vi "Write Error to System Log.vi"(6 "log each error instance (F)":bool, 8 "error in":errorcluster, 10 "message":string, 11 "identifier":string) -> (0 "error out":errorcluster)   [LabVIEW 2020, in "Ballard MIL-STD-1553 Engine.lvlib" / "Custom Device.lvlib"]
uses:
  ca55ed61-c1f5-4d13-8aef-490b87d2cf89.vi
  Custom Device.lvlib
  <vilib>/NI VeriStand/Custom Device Tools/Custom Device Utility Library/Custom Device Utility Library.lvlib
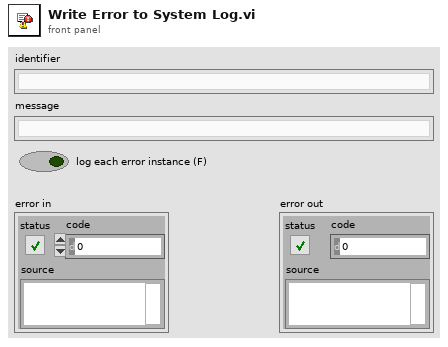
[diagram p1: front panel]
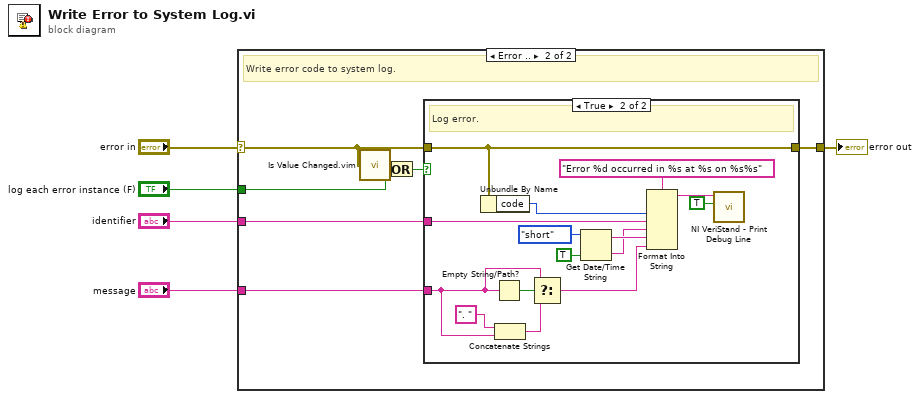
[diagram p0: block diagram]
diagram:
  n1 = case shown="Error .." "error in" {
    selector: "error in" -> [w6 w12]
    tunnel: [w6 w13] -> w5
    tunnel: "log each error instance (F)" -> [_ w9]
    tunnel: "identifier" -> [_ w8]
    tunnel: "message" -> [_ w7]
    frame No Error {
      # "Do not log OK - this is not a heartbeat.\nDo not log warnings."
    }
    frame Error {
      # "Write error code to system log."
      n2 = call "Is Value Changed.vim"("value"=w12) -> ("changed or first call?"=w10:bool)
      n3 = Or(x=w10, y=w9) -> (x .or. y?=w11:bool)
      n4 = case shown="True" w11 {
        tunnel: w12 -> [w14 w23]
        tunnel: [w14 w23] -> w13
        tunnel: w8 -> [_ w22]
        tunnel: w7 -> [_ w19]
        frame False {
          # "Do not log error."
        }
        frame True {
          # "Log error."
          n5 = Unbundle By Name(w23) -> ("code"=w29:i32)
          n6 = Empty String/Path?(string/path=w19) -> (empty?=w21:bool)
          n7 = Concatenate Strings(". ", w19) -> (w18:string)
          n8 = Select(t=w19, s=w21, f=w18) -> (s? t:f=w17:string)
          n9 = Get Date/Time String(date format (0)=enum16{"short", "long", "abbreviated"}."short", want seconds? (F)=TRUE) -> (date string=w16:string, time string=w15:string)  [unwired: 1 in]
          n10 = Format Into String(format string="Error %d occurred in %s at %s on %s%s", w29, w22, w15, w16, w17) -> (resulting string=w27:string)  [unwired: 2 in, 1 out]
          n11 = call <vilib>:"NI VeriStand - Print Debug Line.vi"("Add to log file? (F)"=TRUE, "Message"=w27) -> ()  [unwired: 9 in, 1 out]
        }
      }
    }
  }
  "error out" <- w5
